vi "PH_BeamlineInformation.ProcEvents.vi"(0 "i ref in":refnum<vi>, 5 "error in (no error)":errorcluster) -> (14 "i ref out":refnum<vi>, 19 "error out":errorcluster)   [LabVIEW 2014, in "PH_BeamlineInformation.lvlib"]
doc: "This method is used to define the events the object will listen to. Add your own events here."
uses:
  PH_BeamlineInformation.lvlib
  PH_Beamline_Chief/PH_Beamline_Chief.Section.ctl
  PH_PowerUnit_BaseClass/PH_PowerUnit_BaseClass.PP PU Tags.ctl
  PH_PP_Common/PH_PP_Common.PSU Tags.ctl
  PH_Common/DIM/PH_DIM.Event Declarer.ctl
  CSCore/BaseProcess/BaseProcess.lvlib
  PH_Common/PH_Common.lvlib
  PH_Beamline_Chief/PH_Beamline_Chief.lvlib
  PH_PowerUnit_BaseClass/PH_PowerUnit_BaseClass.lvlib
  PH_PP_Common/PH_PP_Common.lvlib
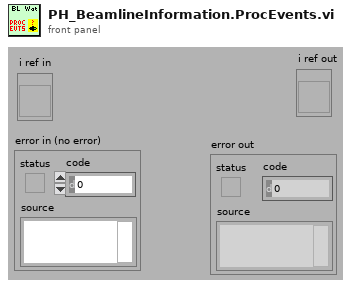
[diagram p1: front panel]
types:
  T1 = typedef "PH_PP_Common.lvlib/PH_PP_Common.PSU Tags.ctl" = enum16{"voltage-indicator", "peak-detect", "current", "voltage", "inihibit-indicator", "end-of-charge", "HV-on-indicator", "overtemperature", "interlock-indicator", "load-fault", "sum-fault", "HV-off-indicator", "DC-ok", "inhibit", "HV-on", "interlock", "reset", "Status", "Limits"}
  T2 = typedef "PH_PowerUnit_BaseClass.lvlib/PH_PowerUnit_BaseClass.PP PU Tags.ctl" = enum16{"Waiting-Time", "PU-in-Use"}
  T3 = typedef "PH_Common.lvlib/PH_DIM.Event Declarer.ctl" = cluster{"Service Name":string, "Selector":string}
  T4 = typedef "PH_Beamline_Chief.lvlib/PH_Beamline_Chief.Section.ctl" = enum16{"None", "YLF", "fs", "fs-YLF", "ns", "PA-Input", "PA-Undelay", "PA-Delay", "PA-before-Bypass", "PA", "PA-Bypass", "PA-Exit", "PA-LL", "LL", "PA-MA", "MA-Exit", "MA-Z6", "Z6", "MA-LB", "LB-TB2", "LB-TB3"}
  T5 = typedef "PH_BeamlineInformation.lvlib/PH_BeamlineInformation.i attribute.ctl" = cluster{"BL GUI Elements of Services":cluster{"Service Name":string, "GUI Elements":refnum<vi>[], "Status":i32}[], "Powermeters":T6, "Efficiency":T7, "Heads":T8[]}
  T6 = typedef "PH_BeamlineInformation.lvlib/PH_BeamlineInformation.Powermeter.ctl" = cluster{"ns FE":cluster{"GUI Ref":refnum<vi>, "Value":dbl}, "fs FE":cluster{"GUI Ref":refnum<vi>, "Value":dbl}, "PA":cluster{"GUI Ref":refnum<vi>, "Value":dbl}, "MA":cluster{"GUI Ref":refnum<vi>, "Value":dbl}, "Z6 green":cluster{"GUI Ref":refnum<vi>, "Value":dbl}, "Z6 IR":cluster{"GUI Ref":refnum<vi>, "Value":dbl}, "Z6 COS":cluster{"GUI Ref":refnum<vi>, "Value":dbl}}
  T7 = typedef "PH_BeamlineInformation.lvlib/PH_BeamlineInformation.Efficiency.ctl" = cluster{"PA Gain":cluster{"GUI Ref":refnum<vi>, "Value":dbl}, "MA Gain":cluster{"GUI Ref":refnum<vi>, "Value":dbl}, "Z6 green Conversion":cluster{"GUI Ref":refnum<vi>, "Value":dbl}, "Z6 Comp Losses":cluster{"GUI Ref":refnum<vi>, "Value":dbl}}
  T8 = typedef "PH_BeamlineInformation.lvlib/PH_BeamlineInformation.Head.ctl" = cluster{"PowerUnit":T9, "in use":cluster{"Value":bool, "GUI Ref":refnum<vi>, "linked":bool}, "voltage":cluster{"Value":dbl, "GUI Ref":refnum<vi>, "linked":bool}}
  T9 = typedef "PH_PP_Common.lvlib/PH_PP_Common.PUs.ctl" = enum16{"no Info", "PA-19mm-1", "PA-19mm-2", "PA-45mm-PILC", "PA-45mm-MAIN", "MA-PU-1", "MA-PU-2", "MA-PU-3", "MA-PU-4", "MA-PU-5", "MA-PU-6", "MA-FR", "MA-PILC", "PA-45mm-DP"}
  T10 = typedef "BaseProcess.lvlib/BaseProcess.event definition.ctl" = cluster{"CAEEvtDef":T11, "Data Descriptor":T12}
  T11 = typedef "CAEObj.lvlib/CAEObj.event definition.ctl" = cluster{"URL":string, "enable":bool, "ignoreResID":bool}
  T12 = typedef "BaseProcess.lvlib/BaseProcess.descriptor string definition.ctl" = string
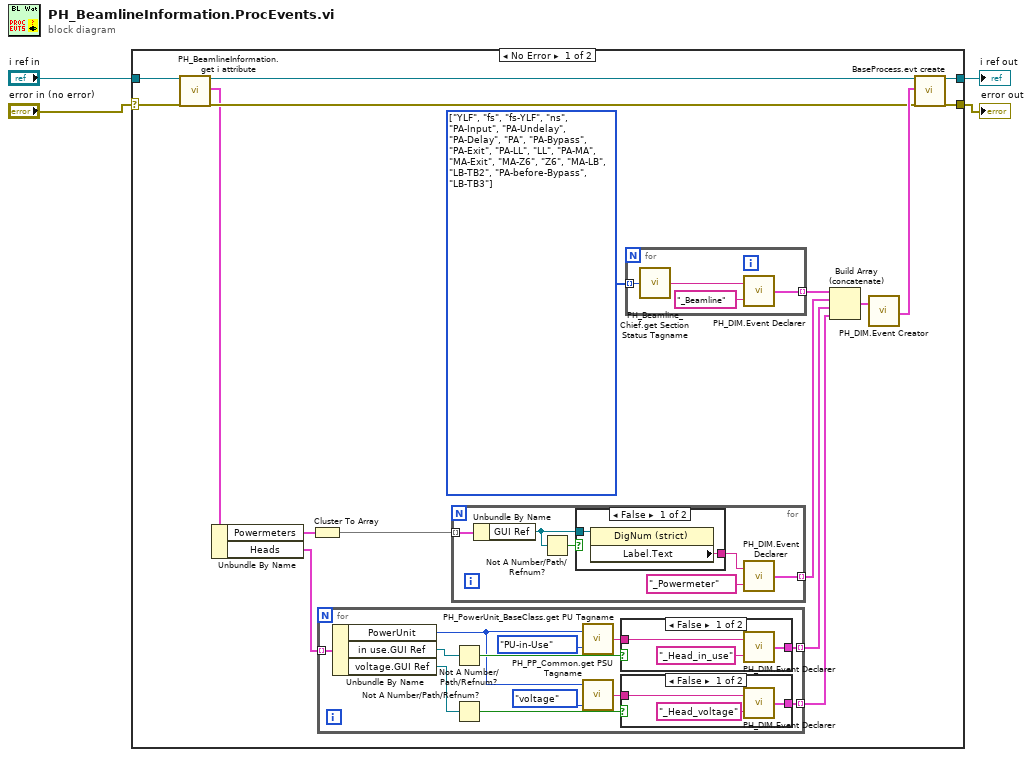
[diagram p0: block diagram]
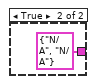
[diagram p2: hidden frame]
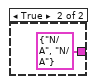
[diagram p3: hidden frame]
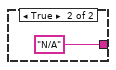
[diagram p4: hidden frame]
diagram:
  n1 = case shown="No Error" "error in (no error)" {
    selector: "error in (no error)" -> [w17 w55]
    tunnel: "i ref in" -> [w15 w56]
    tunnel: [w21 w56] -> w3
    tunnel: [w20 w55] -> w2
    frame No Error {
      w18 = T4[] [enum."YLF", enum."fs", enum."fs-YLF", enum."ns", enum."PA-Input", enum."PA-Undelay", enum."PA-Delay", enum."PA", enum."PA-Bypass", enum."PA-Exit", enum."PA-LL", enum."LL", enum."PA-MA", enum."MA-Exit", enum."MA-Z6", enum."Z6", enum."MA-LB", enum."LB-TB2", enum."PA-before-Bypass", enum."LB-TB3"] items=["None", "YLF", "fs", "fs-YLF", "ns", "PA-Input", "PA-Undelay", "PA-Delay", "PA-before-Bypass", "PA", "PA-Bypass", "PA-Exit", "PA-LL", "LL", "PA-MA", "MA-Exit", "MA-Z6", "Z6", "MA-LB", "LB-TB2", "LB-TB3"]
      n2 = call "PH_BeamlineInformation.get i attribute.vi"("i ref in"=w15, "error in (no error)"=w17) -> ("i ref out"=w14:refnum<vi>, "i attribute"=w13:T5, "error out"=w16:errorcluster)  [unwired: 15 in]
      n3 = Unbundle By Name(w13) -> ("Powermeters"=w12:T6, "Heads"=w5:T8[])
      n4 = Cluster To Array(cluster=w12) -> (array=w9:cluster{"GUI Ref":refnum<vi>, "Value":dbl}[])
      n5 = for {
        tunnel: w5 -> [w32] mode=indexing
        tunnel: [w33] -> w7 mode=indexing
        tunnel: [w27] -> w6 mode=indexing
        n6 = Unbundle By Name(w32) -> ("PowerUnit"=w24:T9, "in use.GUI Ref"=w31:refnum<vi>, "voltage.GUI Ref"=w29:refnum<vi>)
        n7 = Not A Number/Path/Refnum?(number/path/refnum=w31) -> (NaN/Path/Refnum?=w30:bool)
        n8 = Not A Number/Path/Refnum?(number/path/refnum=w29) -> (NaN/Path/Refnum?=w28:bool)
        n9 = call "PH_PowerUnit_BaseClass.get PU Tagname.vi"("PU Tag"=PH_PowerUnit_BaseClass.PP_PU_Tags."PU-in-Use", "PU"=w24) -> ("PU Tagname"=w22:string)
        n10 = call "PH_PP_Common.get PSU Tagname.vi"("PSU Tag"=PH_PP_Common.PSU_Tags."voltage", "PU"=w24) -> ("PSU Tagname"=w23:string)  [unwired: 1 in]
        n11 = case shown="False" w30 {
          tunnel: [w39 T3 {"Service Name"="N/A", "Selector"="N/A"} ("declared DIM Event")] -> w33
          tunnel: w22 -> [w38 _]
          frame False {
            n12 = call "PH_DIM.Event Declarer.vi"("Selector"="_Head_in_use" ("URL"), "Service Name"=w38) -> ("declared DIM Event"=w39:T3)
          }
          frame True {
          }
        }
        n13 = case shown="False" w28 {
          tunnel: [w35 T3 {"Service Name"="N/A", "Selector"="N/A"} ("declared DIM Event")] -> w27
          tunnel: w23 -> [w34 _]
          frame False {
            n14 = call "PH_DIM.Event Declarer.vi"("Selector"="_Head_voltage" ("URL"), "Service Name"=w34) -> ("declared DIM Event"=w35:T3)
          }
          frame True {
          }
        }
      }
      n15 = for {
        tunnel: [w46] -> w10 mode=indexing
        tunnel: w9 -> [w45] mode=indexing
        n16 = Unbundle By Name(w45) -> ("GUI Ref"=w42:refnum<vi>)
        n17 = Not A Number/Path/Refnum?(number/path/refnum=w42) -> (NaN/Path/Refnum?=w43:bool)
        n18 = case shown="False" w43 {
          tunnel: w42 -> [w49 _]
          tunnel: [w48 "N/A" ("Label.Text")] -> w44
          frame False {
            n19 = property class="DigNum (strict)"(reference=w49) -> ("Label.Text"=w48:string)  [unwired: 1 in, 2 out]
          }
          frame True {
          }
        }
        n20 = call "PH_DIM.Event Declarer.vi"("Selector"="_Powermeter" ("URL"), "Service Name"=w44) -> ("declared DIM Event"=w46:T3)
      }
      n21 = for {
        tunnel: [w53] -> w8 mode=indexing
        tunnel: w18 -> [w51] mode=indexing
        n22 = call "PH_Beamline_Chief.get Section Status Tagname.vi"("Beamline Section"=w51) -> ("Section Status Tagname"=w52:string)
        n23 = call "PH_DIM.Event Declarer.vi"("Selector"="_Beamline" ("string"), "Service Name"=w52) -> ("declared DIM Event"=w53:T3)
      }
      n24 = Build Array (concatenate)(w8, w10, w7, w6) -> (w11:T3[])
      n25 = call "PH_DIM.Event Creator.vi"("Trendmessage Services"=w11) -> ("DIM Service Events"=w19:T10[])  [unwired: 18 in]
      n26 = call "BaseProcess.evt create.vi"("i ref in"=w14, "newEvents"=w19, "error in (no error)"=w16) -> ("i ref out"=w21:refnum<vi>, "error out"=w20:errorcluster)  [unwired: 13 in, 2 out]
    }
    frame Error {
    }
  }
  "i ref out" <- w3
  "error out" <- w2
